vi "1. Термометр.vi"() -> ()   [LabVIEW 2020]
panel:
  out "Numeric2":dbl
  out "Numeric":dbl
  out "Температура в градусах Реамюра, R":dbl(slide) scale=0.0..21.0
  out "Температура в градусах Фаренгейта, F":dbl(slide) scale=0.0..78.0
  in  "Регулировка выходного напряжения\n датчика температуры, В":dbl(knob) scale=0.0..23.0
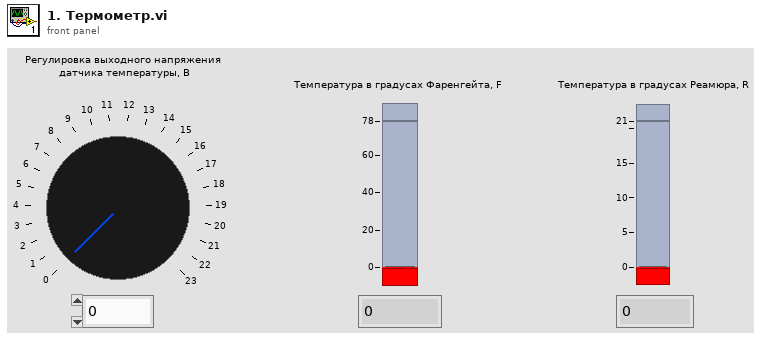
[diagram p1: front panel]
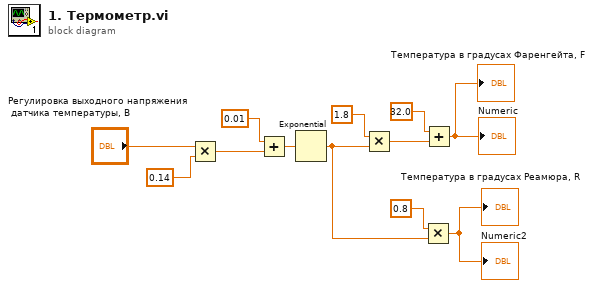
[diagram p0: block diagram]
diagram:
  n1 = Multiply(x="Регулировка выходного напряжения\n датчика температуры, В", y=0.14) -> (x*y=w9:dbl)
  n2 = Add(x=0.01, y=w9) -> (x+y=w8:dbl)
  n3 = Exponential(1:w8) -> (0:w2:dbl)
  n4 = Multiply(x=1.8, y=w2) -> (x*y=w6:dbl)
  n5 = Multiply(x=0.8, y=w2) -> (x*y=→"Температура в градусах Реамюра, R" →"Numeric2":dbl)
  n6 = Add(x=32.0, y=w6) -> (x+y=→"Температура в градусах Фаренгейта, F" →"Numeric":dbl)
